vi "Read_Encoders.vi"(8 "error in (no error)":errorcluster, 10 "Cluster in":T1={FALSE, "Tick Count(uSec)"=0, "Counter Value"=[0, 0, 0, 0], "x-y"=[0, 0, 0, 0]}, 11 "Reset Encoders":bool) -> (0 "error out":errorcluster, 1 "Cluster Out":T1, 2 "Updated":bool, 3 "Tick Count(uSec)":u32 caption="Tick Count(Ticks)", 5 "output cluster":T2)   [LabVIEW 2018]
uses:
  <vilib>/Studica/Studica Toolkit/Background/Mxp Selection.ctl
  <vilib>/rvi/Arithmetic/AddSubMult/XNode/nirviSatArithmetic.xnode
panel:
  out "appended array":i64[](array[numeric])
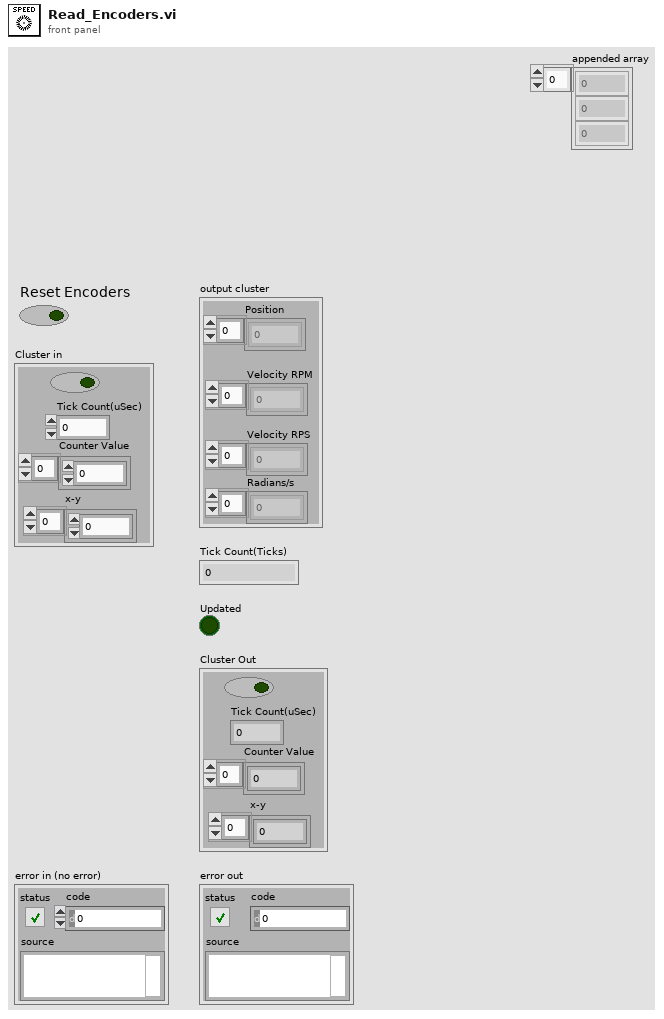
[diagram p1: front panel]
types:
  T1 = cluster{bool, "Tick Count(uSec)":u32, "Counter Value":i32[], "x-y":i32[]}
  T2 = cluster{"Position":i32[], "Velocity RPM":dbl[], "Velocity RPS":dbl[], "Radians/s":dbl[]}
  T3 = typedef "Mxp Selection.ctl" = enum16{"MXP A", "MXP B"}
  T4 = cluster{"Counter Value":dbl[], dbl[], dbl[], dbl[]}
  T5 = cluster{bool, "Tick Count(uSec)":u32, "Counter Value":dbl[], "x-y":dbl[]}
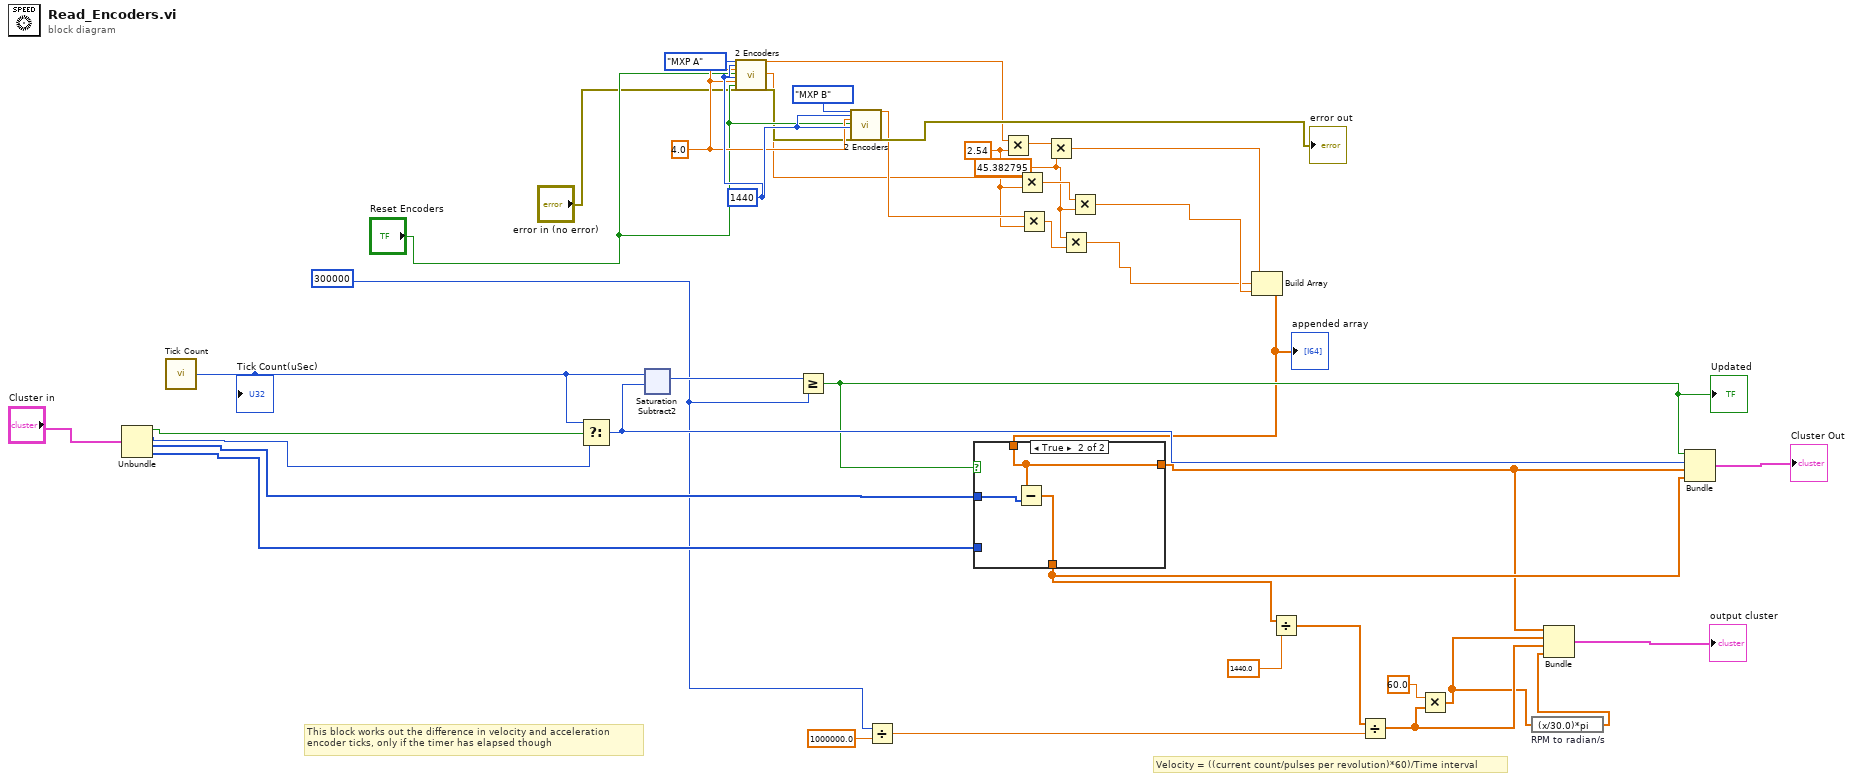
[diagram p0: block diagram]
diagram:
  w5 = 45.382795 ("y")
  w41 = 4.0 ("Wheel Diameter M1 (inches)")
  w42 = u32 1440 ("Ticks Per Rev M0")
  w31 = 2.54 ("y")
  w8 = 300000
  # "Velocity = ((current count/pulses per revolution)*60)/Time interval"
  # "This block works out the difference in velocity and acceleration \nencoder ticks, only if the timer has elapsed though"
  n1 = Unbundle("Cluster in") -> (w15:bool, "Tick Count(uSec)"=w14:u32, "Counter Value"=w13:i32[], "x-y"=w12:i32[])
  n2 = call "Tick Count"() -> ("Tick Count(uSec)"=w24:u32)
  "Tick Count(uSec)" <- w24
  n3 = Select(t=w24, s=w15, f=w14) -> (s? t:f=w23:u32)
  n4 = xnode ("Saturation Subtract2")("x"=w24, "y"=w23) -> ("x-y"=w19:u32)
  n5 = call <vilib>:"2 Encoders.vi"("Mxp Side"=Mxp_Selection."MXP A", "Ticks Per Rev M0"=w42, "Wheel Diameter M0 (inches)"=w41, "Reset Encoder 0"="Reset Encoders", "Ticks Per Rev M1"=w42, "Wheel Diameter M1 (inches)"=w41, "Reset Encoder 1"="Reset Encoders", "error in (no error)"="error in (no error)") -> ("Distance M0 (inches)"=w32:dbl, "Distance M1 (inches)"=w33:dbl, "error out"=w36:errorcluster)  [unwired: 17 in]
  n6 = Greater Or Equal?(x=w19, y=w8) -> (x >= y?=w22:bool)
  "Updated" <- w22
  n7 = call <vilib>:"2 Encoders.vi"("Mxp Side"=Mxp_Selection."MXP B", "Ticks Per Rev M0"=w42, "Wheel Diameter M0 (inches)"=w41, "Reset Encoder 0"="Reset Encoders", "Ticks Per Rev M1"=w42, "error in (no error)"=w36) -> ("Distance M0 (inches)"=w34:dbl, "error out"=→"error out":errorcluster)  [unwired: 19 in, 1 out]
  n8 = Divide(x=w8, y=1000000.0) -> (x/y=w26:dbl)
  n9 = Multiply(x=w32, y=w31) -> (x*y=w7:dbl)
  n10 = Multiply(x=w33, y=w31) -> (x*y=w6:dbl)
  n11 = Multiply(x=w34, y=w31) -> (x*y=w4:dbl)
  n12 = Multiply(x=w7, y=w5) -> (x*y=w3:dbl)
  n13 = Multiply(x=w5, y=w4) -> (x*y=w1:dbl)
  n14 = Multiply(x=w6, y=w5) -> (x*y=w2:dbl)
  n15 = Build Array(w3, w1, w2) -> (w18:dbl[])
  "appended array" <- w18
  n16 = case shown="True" w22 {
    tunnel: w13 -> [w43 w47]
    tunnel: [w44 w46] -> w27
    tunnel: w12 -> [w44 _]
    tunnel: [w43 w45] -> w25
    tunnel: w18 -> [_ w45]
    frame False {
    }
    frame True {
      n17 = Subtract(x=w45, y=w47) -> (x-y=w46:dbl[])
    }
  }
  n18 = Divide(x=w27, y=1440.0) -> (x/y=w28:dbl[])
  n19 = Divide(x=w28, y=w26) -> (x/y=w29:dbl[])
  n20 = Multiply(x=60.0 ("y"), y=w29) -> (x*y=w11:dbl[])
  n21 = expression code="(x/30.0)*pi" "RPM to radian/s"(w11) -> (w10:dbl[])
  n22 = Bundle("Counter Value"=w25, w11, w29, w10) -> (→"output cluster":T4)  [unwired: 1 in]
  n23 = Bundle(w22, "Tick Count(uSec)"=w23, "Counter Value"=w25, "x-y"=w27) -> (→"Cluster Out":T5)  [unwired: 1 in]
